vi "sensor de temperatura y ir emisor.vi"() -> ()   [LabVIEW 2026]
uses:
  <vilib>/Instr/_visa.llb/VISA Configure Serial Port (Instr).vi
panel:
  out "Temperatura °C":dbl(knob) scale=0.0..100.0
  in  "Stop Button":bool
  out "?":bool
  in  "IR EMISSION":bool
  out "Temperatura °C":dbl(slide) scale=0.0..100.0
  out "Bajo":bool
  out "normal":bool
  out "Alto":bool
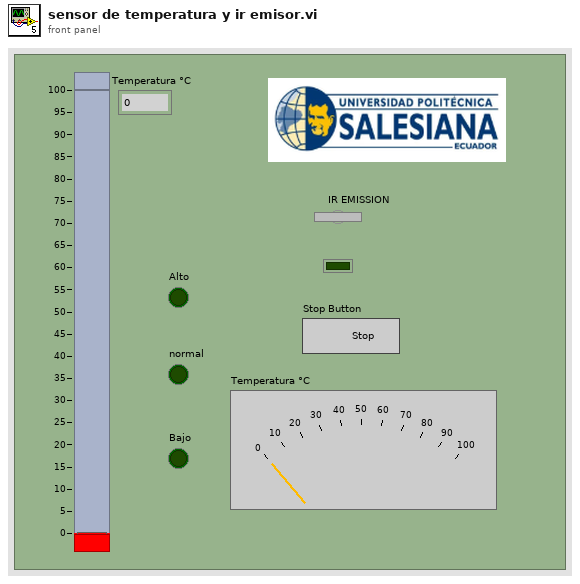
[diagram p1: front panel]
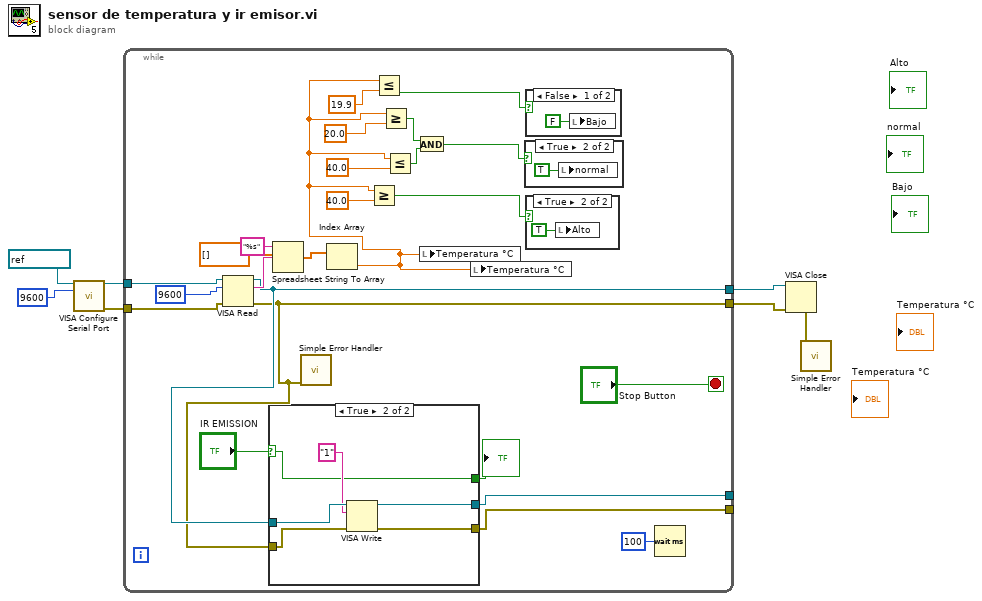
[diagram p0: block diagram]
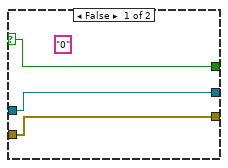
[diagram p2: hidden frame]
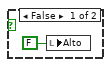
[diagram p3: hidden frame]
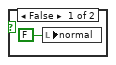
[diagram p4: hidden frame]
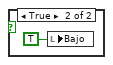
[diagram p5: hidden frame]
diagram:
  n1 = call-poly "VISA Configure Serial Port"("VISA resource name"=refnum<visa-resource-name> "COM4", "baud rate (9600)"=u32 9600) -> ("VISA resource name out"=w5:refnum<visa-resource-name>, "error out"=w7:errorcluster)  [unwired: 12 in]
  n2 = while {
    tunnel: w7 -> [w16]
    tunnel: [w13] -> w6
    tunnel: w5 -> [w17]
    tunnel: [w14] -> w4
    tunnel: [w12] -> _
    tunnel: [w11] -> _
    stop <- "Stop Button" stop-if-true
    n3 = VISA Read(VISA resource name=w17, byte count=u32 9600 ("baud rate (9600)"), error in (no error)=w16) -> (VISA resource name out=w14:refnum<visa-resource-name>, read buffer=w31:string, error out=w13:errorcluster)  [unwired: 1 out]
    n4 = case shown="True" "IR EMISSION" {
      selector: "IR EMISSION" -> [w35 w36]
      tunnel: [w35 w36] -> w10
      tunnel: w14 -> [w34 w41]
      tunnel: w13 -> [w33 w40]
      tunnel: [w34 w38] -> w12
      tunnel: [w33 w37] -> w11
      frame False {
        (unwired) "0"
      }
      frame True {
        n5 = VISA Write(VISA resource name=w41, write buffer="1", error in (no error)=w40) -> (VISA resource name out=w38:refnum<visa-resource-name>, error out=w37:errorcluster)  [unwired: 1 out]
      }
    }
    "?" <- w10
    n6 = Spreadsheet String To Array(format string="%s", spreadsheet string=w31, array type (2D Dbl)=dbl[] []) -> (array=w28:dbl[])  [unwired: 1 in]
    n7 = call <vilib>:"Simple Error Handler.vi"("error in (no error)"=w13) -> ()  [unwired: 4 in, 5 out]
    n8 = Index Array(array=w28) -> (element=w9:dbl)  [unwired: 1 in]
    n9 = Greater Or Equal?(x=w9, y=40.0) -> (x >= y?=w22:bool)
    n10 = Less Or Equal?(x=w9, y=19.9) -> (x <= y?=w19:bool)
    n11 = Greater Or Equal?(x=w9, y=20.0) -> (x >= y?=w24:bool)
    n12 = Less Or Equal?(x=w9, y=40.0) -> (x <= y?=w23:bool)
    n13 = And(x=w24, y=w23) -> (x .and. y?=w27:bool)
    n14 = local write "Temperatura °C"(w9) -> ()
    n15 = local write "Temperatura °C"(w9) -> ()
    n16 = case shown="True" w27 {
      frame False {
        n17 = local write "normal"(FALSE ("normal")) -> ()
      }
      frame True {
        n18 = local write "normal"(TRUE ("normal")) -> ()
      }
    }
    n19 = case shown="False" w19 {
      frame False {
        n20 = local write "Bajo"(FALSE ("Bajo")) -> ()
      }
      frame True {
        n21 = local write "Bajo"(TRUE ("Bajo")) -> ()
      }
    }
    n22 = case shown="True" w22 {
      frame False {
        n23 = local write "Alto"(FALSE ("Alto")) -> ()
      }
      frame True {
        n24 = local write "Alto"(TRUE ("Alto")) -> ()
      }
    }
    n25 = Wait (ms)(milliseconds to wait=u32 100) -> ()  [unwired: 1 out]
  }
  n26 = VISA Close(VISA resource name=w4, error in (no error)=w6) -> (error out=w3:errorcluster)
  n27 = call <vilib>:"Simple Error Handler.vi"("error in (no error)"=w3) -> ()  [unwired: 4 in, 5 out]
